vi "Function Generator with FM.vi"() -> ()   [LabVIEW 2023]
doc: "This example demonstrates how to simulate a Frequency Modulation (FM) using the signal generation functions. This VI also presents the Power Spectrum of the FM signal."
uses:
  <vilib>/measure/maspectr.llb/FFT Power Spectrum and PSD for 1 Chan.vi
  <vilib>/measure/NI_MABase.lvlib
  <vilib>/measure/NI_MAPro.lvlib
panel:
  in  "Carrier Frequency (Hz)":dbl(knob)=205410.22592152198 min=86453.20197044335 scale=22413.793103448275..1000000.0 scale format="%#_6p"
  in  "FM Deviation (Hz)":dbl(slide)=154517.79084245834 scale=1.0..205410.22592152198 scale format="%#_6p"
  in  "Baseband Signal":T1(ring)
  in  "Baseband Frequency (Hz)":dbl(knob)=22413.793103448275 scale=1.0..100000.0 scale format="%#_6p"
  in  "Tab Control":T2(tab)
  out "Baseband Graph":waveform(dbl)(graph)
  out "Carrier Graph":waveform(dbl)(graph)
  out "Power Spectrum":cluster{"f0":dbl, "df":dbl, "magnitude":dbl[]}(graph)
  out "Demodulated and filtered Signal":waveform(dbl)[](graph)
  in  "Stop":bool
  # "Simulating a Frequency Modulation (FM) Signal"
  # "Overview: \nFrequency Modulation (FM) is a form of modulation in which changes to the frequency of the carrier wave correspond directly with changes in the baseband signal. This is considered an analog form of modulation because the baseband signal is typically an analog waveform without discrete, digital values.\n\nThe basic principle behind FM modulation is that the amplitude of an analog baseband signal can be represented by a slightly different frequency of the carrier.\n\nInstructions: \n1. Run the VI.\n2. Change the Baseband Frequency (Hz) and the Baseband Signal and see how it affects the Baseband Graph on the Input Signals tab. Also, modify the Carrier Frequency (Hz) and see how that affects the Carrier Graph.\n3. Go to the FM Modulated Signal tab and verify the resulting Demodulated and filtered Signal and the Power Spectrum of the signal. Change the Baseband Frequency and Carrier frequency again to study the resulting signal. Modify the FM Deviation (Hz) and see how that affects the Power Spectrum.\n4. Click Stop to stop the VI."
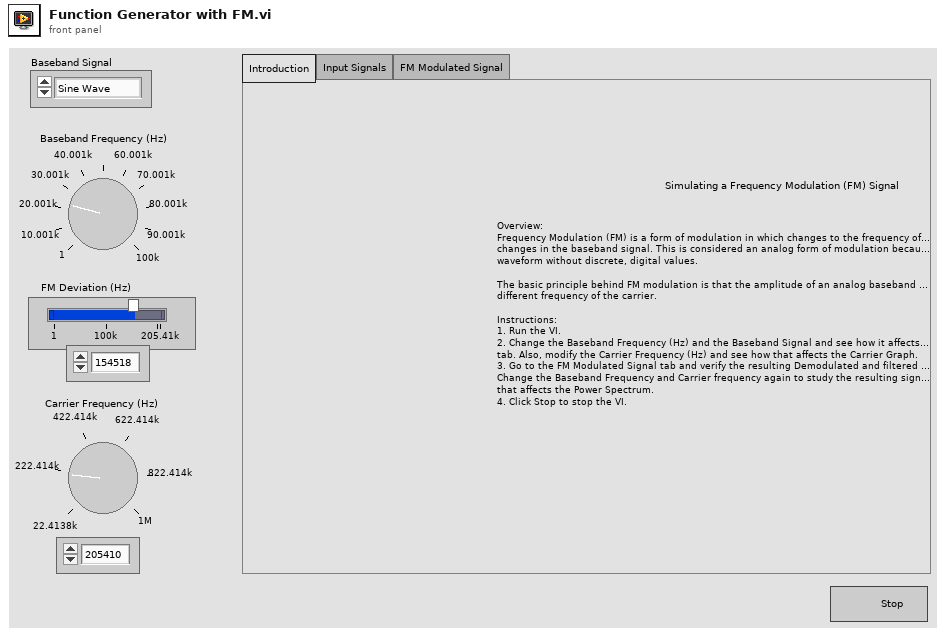
[diagram p1: front panel]
types:
  T1 = enum16{"Sine Wave", "Triangle Wave", "Square Wave", "Sawtooth Wave"}
  T2 = enum32{"Introduction", "Input Signals", "FM Modulated Signal"}
  T3 = cluster{"Sampling frequency (samples/sec)":dbl, "Sampling frequency (samples/sec)":dbl}
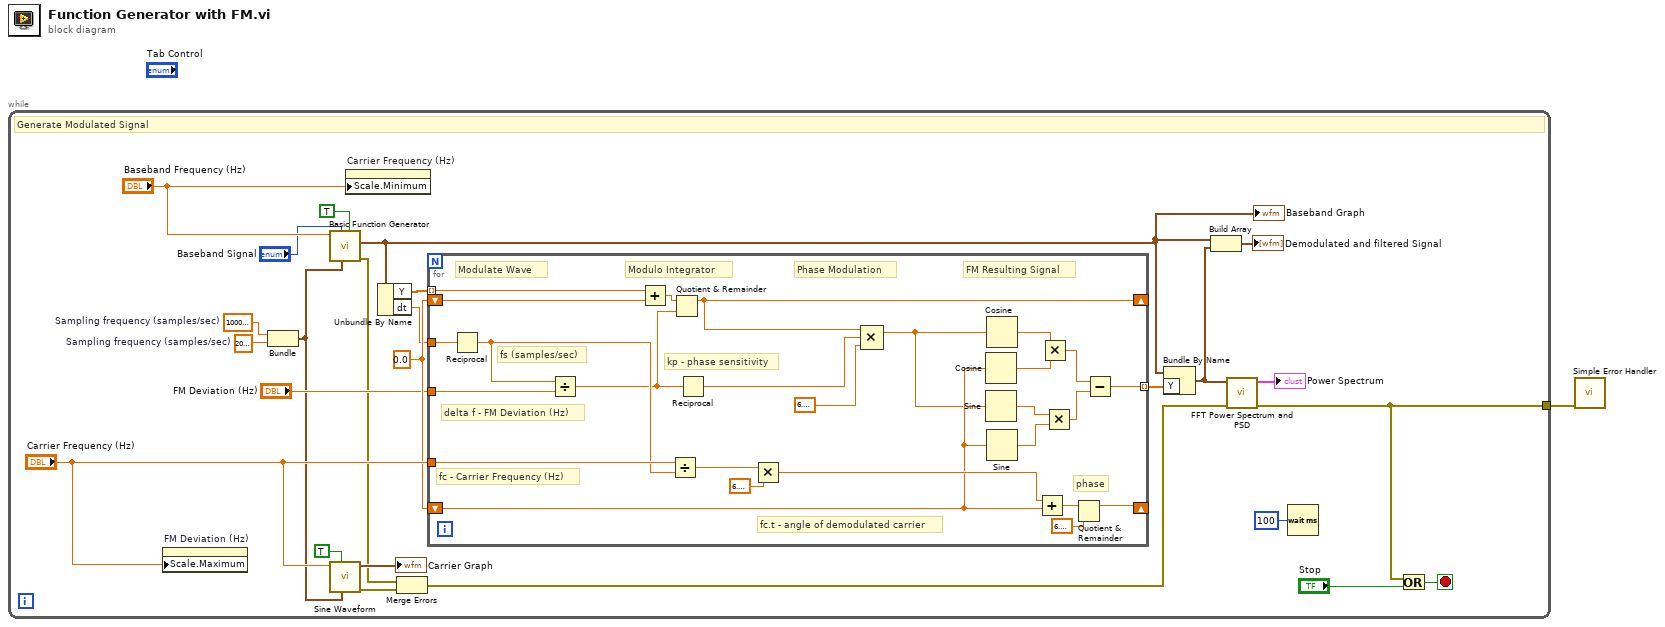
[diagram p0: block diagram]
diagram:
  n1 = while {
    tunnel: [w2] -> w1
    stop <- w3 stop-if-true
    w8 = 2000.0  # Sampling frequency (samples/sec)
    w24 = 0.0
    w21 = 10000000.0  # Sampling frequency (samples/sec)
    # "Generate Modulated Signal"
    n2 = property on="FM Deviation (Hz)" class="Slide (strict)"("Scale.Maximum"="Carrier Frequency (Hz)") -> ()  [unwired: 2 in, 2 out]
    n3 = Bundle("Sampling frequency (samples/sec)"=w21, "Sampling frequency (samples/sec)"=w8) -> (w7:T3)  [unwired: 1 in]
    n4 = call <vilib>:"Basic Function Generator.vi"("reset signal"=TRUE, "sampling info"=w7, "signal type"="Baseband Signal", "frequency"="Baseband Frequency (Hz)") -> ("error out"=w5:errorcluster, "signal out"=w12:waveform(dbl))  [unwired: 5 in, 1 out]
    "Baseband Graph" <- w12
    n5 = call <vilib>:"Sine Waveform.vi"("sampling info"=w7, "reset signal"=TRUE, "frequency"="Carrier Frequency (Hz)") -> ("error out"=w6:errorcluster, "signal out"=→"Carrier Graph":waveform(dbl))  [unwired: 7 in]
    n6 = property on="Carrier Frequency (Hz)" class="Knob (strict)"("Scale.Minimum"="Baseband Frequency (Hz)") -> ()  [unwired: 2 in, 2 out]
    n7 = Unbundle By Name(w12) -> ("Y"=w17:dbl[], "dt"=w20:dbl)
    n8 = Merge Errors(w5, w6) -> (w4:errorcluster)
    n9 = for {
      tunnel: w20 -> [w52]
      tunnel: "FM Deviation (Hz)" -> [w51]
      shift-right: [w38] -> _
      shift-left: w24 -> [w37]
      tunnel: w17 -> [w36] mode=indexing
      tunnel: "Carrier Frequency (Hz)" -> [w50]
      tunnel: [w45] -> w19 mode=indexing
      shift-right: [w41] -> _
      shift-left: w24 -> [w34]
      # "fc.t - angle of demodulated carrier"
      # "Modulate Wave"
      # "fc - Carrier Frequency (Hz)"
      # "delta f - FM Deviation (Hz)"
      # "phase"
      # "FM Resulting Signal"
      # "Phase Modulation"
      # "kp - phase sensitivity"
      # "Modulo Integrator"
      # "fs (samples/sec)"
      n10 = Reciprocal(x=w52) -> (1/x=w49:dbl)
      n11 = Divide(x=w49, y=w51) -> (x/y=w39:dbl)
      n12 = Add(x=w36, y=w37) -> (x+y=w40:dbl)
      n13 = Divide(x=w50, y=w49) -> (x/y=w47:dbl)
      n14 = Quotient & Remainder(x=w40, y=w39) -> (x-y*floor(x/y)=w38:dbl)  [unwired: 1 out]
      n15 = Reciprocal(x=w39) -> (1/x=w28:dbl)
      n16 = Multiply(x=w47, y=6.283185307179586) -> (x*y=w44:dbl)
      n17 = Compound Arithmetic op=MULTIPLY(w38, w28, 6.283185307179586) -> (w29:dbl)
      n18 = Cosine(x=w34) -> (cos(x)=w31:dbl)
      n19 = Sine(x=w29) -> (sin(x)=w30:dbl)
      n20 = Cosine(x=w29) -> (cos(x)=w32:dbl)
      n21 = Sine(x=w34) -> (sin(x)=w33:dbl)
      n22 = Add(x=w44, y=w34) -> (x+y=w43:dbl)
      n23 = Multiply(x=w32, y=w31) -> (x*y=w46:dbl)
      n24 = Multiply(x=w30, y=w33) -> (x*y=w35:dbl)
      n25 = Quotient & Remainder(x=w43, y=6.283185307179586) -> (x-y*floor(x/y)=w41:dbl)  [unwired: 1 out]
      n26 = Subtract(x=w46, y=w35) -> (x-y=w45:dbl)
    }
    n27 = Bundle By Name(cluster=w12, "Y"=w19) -> (w10:waveform(dbl))
    n28 = Build Array(w12, w10) -> (→"Demodulated and filtered Signal":waveform(dbl)[])
    n29 = call-poly <vilib>:"FFT Power Spectrum and PSD.vi"("error in (no error)"=w4, "time signal"=w10) -> ("error out"=w2:errorcluster, "Power Spectrum / PSD"=→"Power Spectrum":cluster{"f0":dbl, "df":dbl, "magnitude":dbl[]})  [unwired: 6 in, 2 out]
    n30 = Wait (ms)(milliseconds to wait=u32 100) -> ()  [unwired: 1 out]
    n31 = Or(x=w2, y="Stop") -> (x .or. y?=w3:bool)
  }
  n32 = call <vilib>:"Simple Error Handler.vi"("error in (no error)"=w1) -> ()  [unwired: 4 in, 5 out]
